vi "Shutdown.vi"(8 "error in":errorcluster, 11 "ELAN Master in":refnum<class "ELAN Master.lvclass">) -> (0 "error out":errorcluster)   [LabVIEW 2021, in "ELAN Master.lvclass"]
doc: "This provides an interface for the master to close a connection to the slave."
uses:
  ELAN Master.lvclass
  ELAN Master.lvclass/ELAN Master.ctl
  Transmission Data Unit/ELAN/ELAN Data Unit.lvclass/ELAN Data Unit.ctl
  Transmission Data Unit/ELAN/ELAN Data Unit.lvclass
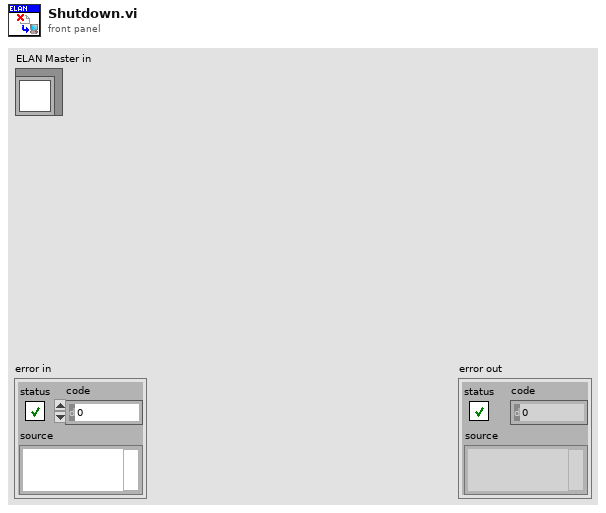
[diagram p1: front panel]
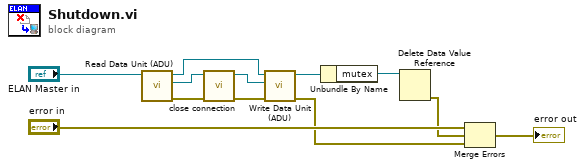
[diagram p0: block diagram]
diagram:
  n1 = call "Read Data Unit (ADU).vi"("ELAN Master in"="ELAN Master in") -> ("error out"=w10:errorcluster, "ASCII Data Unit"=w9:refnum<class "ELAN Data Unit.lvclass">, "ELAN Master out"=w5:refnum<class "ELAN Master.lvclass">)  [unwired: 8 in]
  n2 = call "close connection.vi"("error in"=w10, "ELAN data unit (ADU) in"=w9) -> ("error out"=w6:errorcluster, "ELAN data unit (ADU) out"=w7:refnum<class "ELAN Data Unit.lvclass">)  [unwired: 8 in]
  n3 = call "Write Data Unit (ADU).vi"("error in (no error)"=w6, "ASCII Data Unit"=w7, "ELAN Master in"=w5) -> ("error out"=w1:errorcluster, "ELAN Master out"=w4:refnum<class "ELAN Master.lvclass">)  [unwired: 7 in]
  n4 = Unbundle By Name(w4) -> ("mutex"=w11:refnum<data-value>)
  n5 = Delete Data Value Reference(data value reference=w11) -> (error out=w2:errorcluster)  [unwired: 1 in, 1 out]
  n6 = Merge Errors("error in", w2, w1) -> (→"error out":errorcluster)
